vi "TEST_Setup_ExcitsEjects.vi"() -> ()   [LabVIEW 2017]
uses:
  controls/EXCIT_Form_Selector.ctl
  controls/EXCIT_Table.ctl
panel:
  in  "EXCIT Table":T1={"Number of Excits"=0, "Number of Ejects"=0, "Sampling Frequency"=0.0, "Waveforms Table"=[["Excit1", "name", "Swift", "0.5", "1200", "70", "150", "550", "0", "0", "0"]]}
  out "Variant out":variant
  in  "Variant":variant
  out "error out":errorcluster caption="sortie d'erreur"
  in  "error in (no error)":errorcluster
  in  "Excit Form":T2=enum."Swift"
  out "Excitation Signal":T3(graph)
  in  "Fs":dbl=1.0 caption="Sampling Frequency (MHz)" min=1.0 max=100.0
  out "Wfm table":cluster{"Excits Table":string[][]}
  in  "Excit Sandbox":i32(listbox)
  in  "Ejects":u32
  in  "Excits":u32
  in  "Generate":bool
  in  "Update":bool
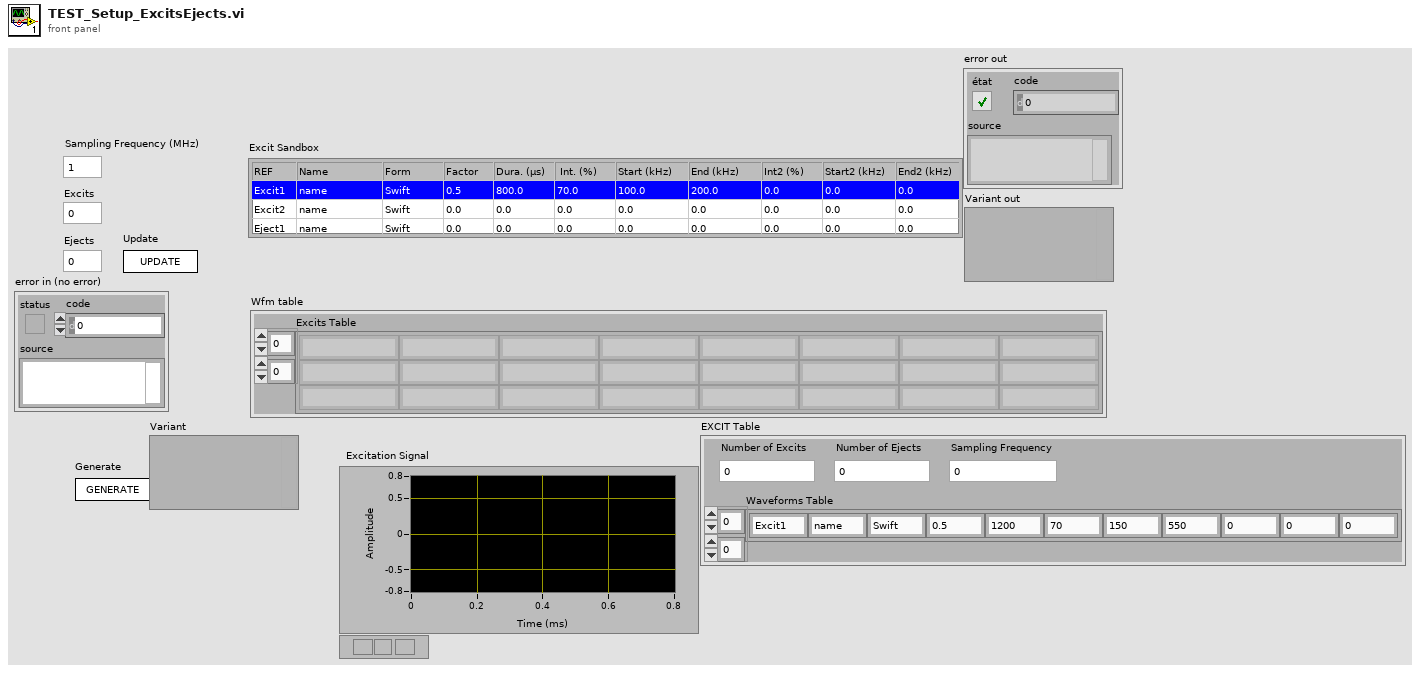
[diagram p1: front panel]
types:
  T1 = typedef "EXCIT_Table.ctl" = cluster{"Number of Excits":u16, "Number of Ejects":u16, "Sampling Frequency":dbl, "Waveforms Table":string[][]}
  T2 = typedef "EXCIT_Form_Selector.ctl" = enum16{"Sinus", "Chirp", "Swift", "TwoSwift", "Ramp"}
  T3 = cluster{"X Time":dbl[], "Signal Excitation":dbl[]}
  T4 = enum16{"Sinus", "Chirp", "Swift", "TwoSwift", "Ramp"}
  T5 = typedef "LVRowAndColumnTypeDef.ctl" = cluster{"Row":i32, "Column":i32}
  T6 = typedef "LVPoint32TypeDef.ctl" = cluster{"Horizontal":i32, "Vertical":i32}
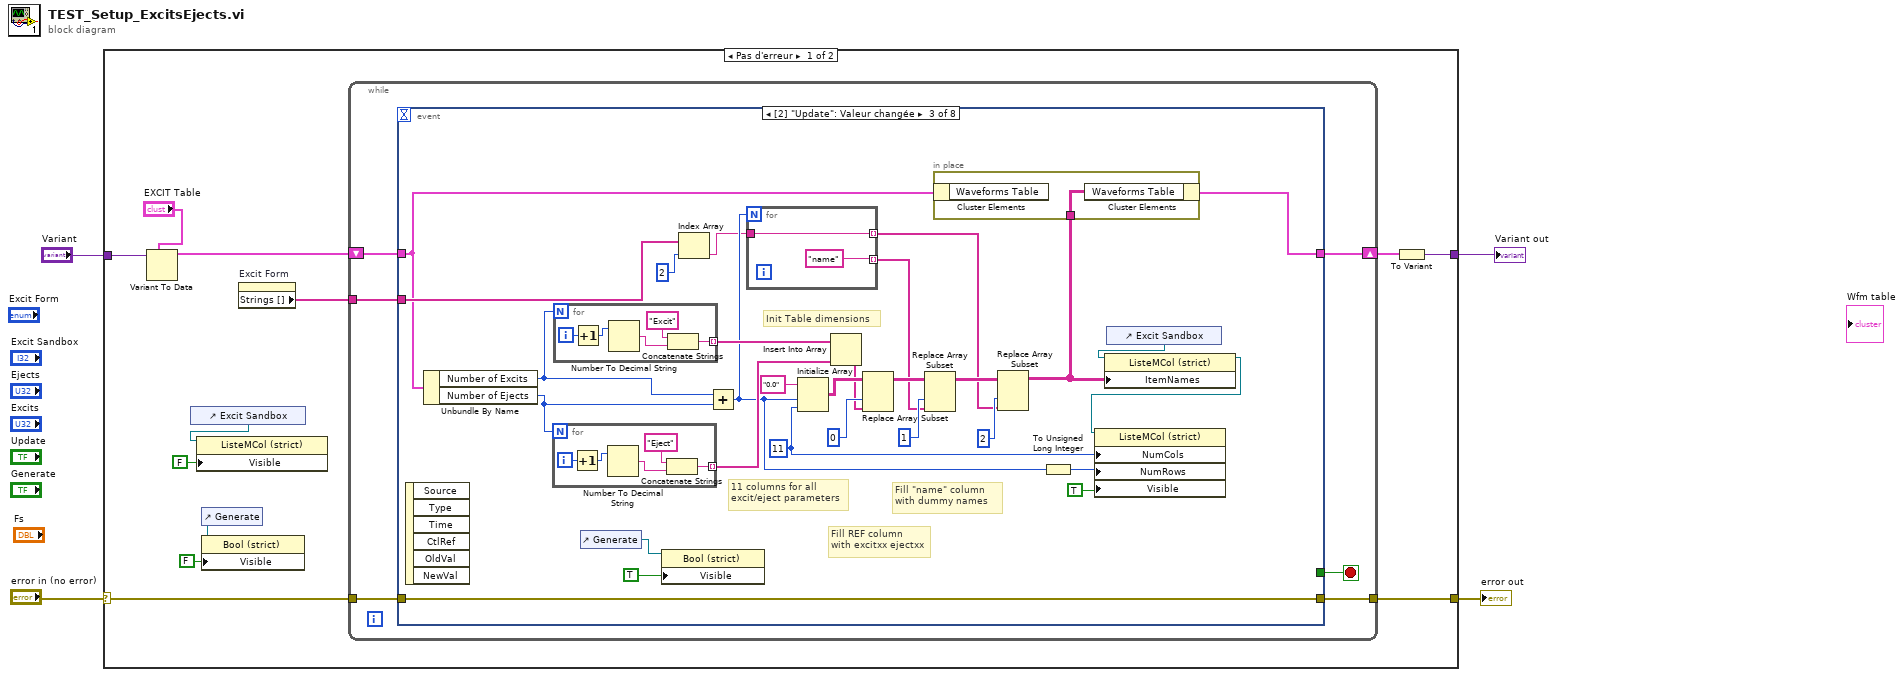
[diagram p0: block diagram]
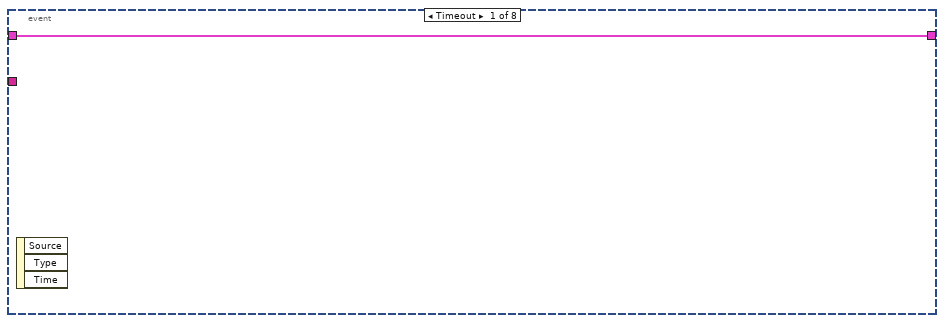
[diagram p2: hidden frame]
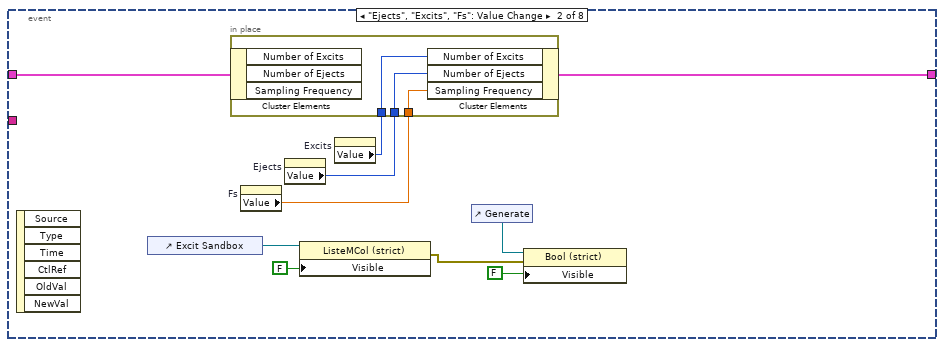
[diagram p3: hidden frame]
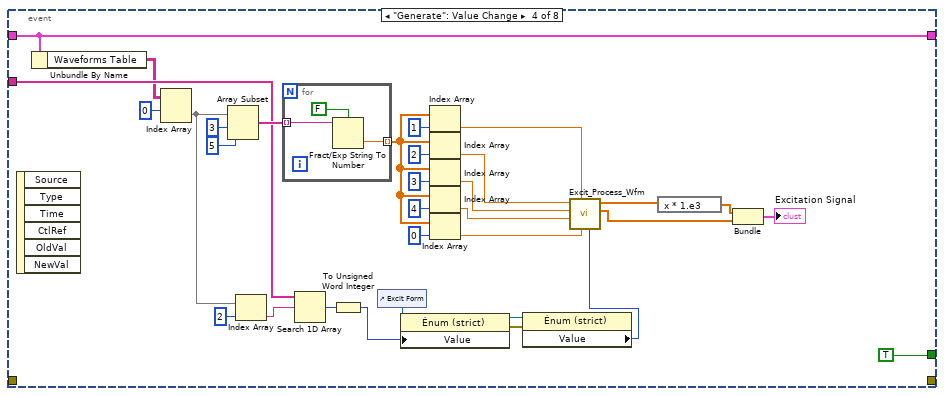
[diagram p4: hidden frame]
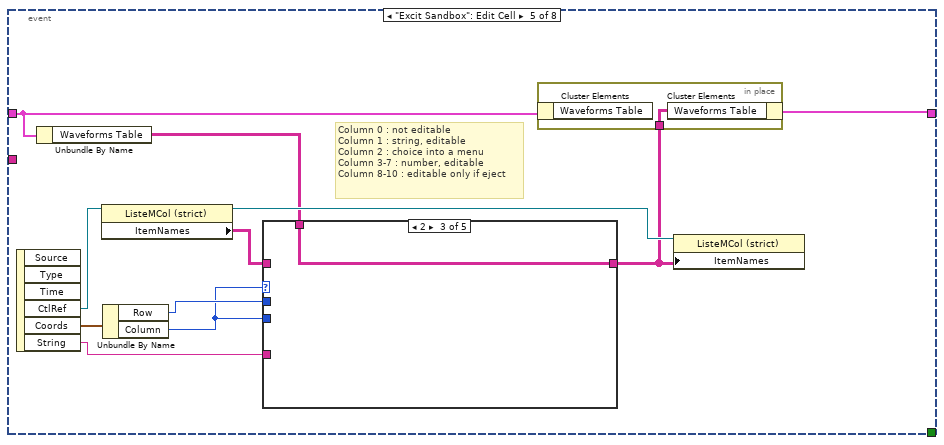
[diagram p5: hidden frame]
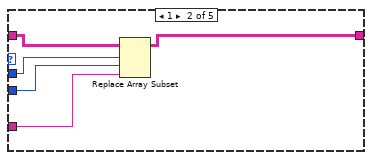
[diagram p7: hidden frame]
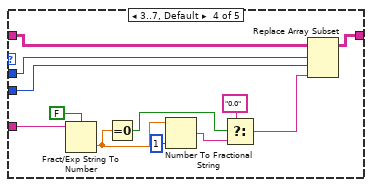
[diagram p8: hidden frame]
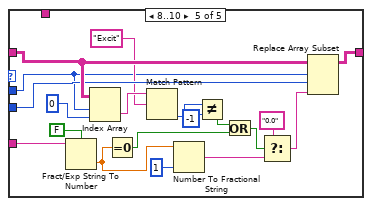
[diagram p9: hidden frame]
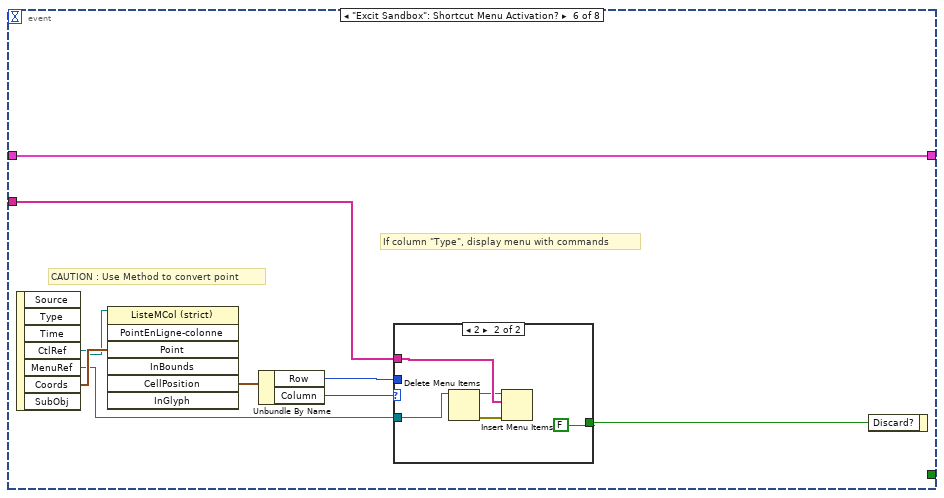
[diagram p10: hidden frame]
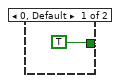
[diagram p11: hidden frame]
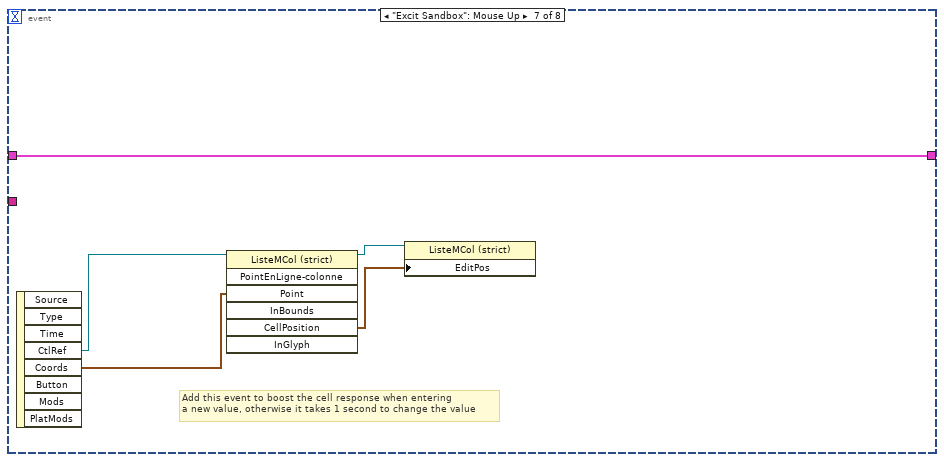
[diagram p12: hidden frame]
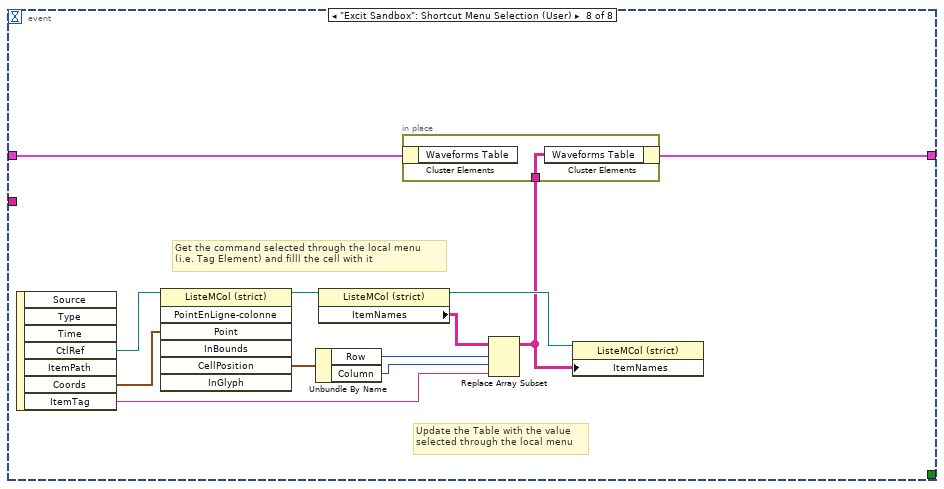
[diagram p13: hidden frame]
diagram:
  n1 = case shown="Pas d'erreur" "error in (no error)" {
    selector: "error in (no error)" -> [w6 _]
    tunnel: "Variant" -> [w11 _]
    tunnel: [w7 _] -> w2
    tunnel: [w5 _] -> w1
    frame No Error {
      n2 = Variant To Data(type="EXCIT Table", Variant=w11) -> (data=w9:T1)  [unwired: 1 in, 1 out]
      n3 = control-ref of="Excit Sandbox"() -> (w14:refnum<vi>)
      n4 = property class="ListeMCol (strict)"(reference=w14, "Visible"=FALSE) -> ()  [unwired: 1 in, 2 out]
      n5 = control-ref of="Generate"() -> (w16:refnum<vi>)
      n6 = property class="Bool (strict)"(reference=w16, "Visible"=FALSE) -> ()  [unwired: 1 in, 2 out]
      n7 = property on="Excit Form" class="Énum (strict)"() -> ("Strings []"=w12:string[])  [unwired: 2 in, 2 out]
      n8 = while {
        tunnel: w12 -> [w21]
        shift-right: [w19] -> w8
        shift-left: w9 -> [w20]
        tunnel: w6 -> [w18]
        tunnel: [w17] -> w5
        stop <- w22 stop-if-true
        n9 = event shown="[2] \"Update\": Valeur changée" {
          selector: _ -> [_ _ _ _ _ _ _ _]
          dyn-events: _ -> [_ _ _ _ _ _ _ _]
          timeout: _ -> [_ _ _ _ _ _ _ _]
          tunnel: [_ _ _ TRUE _ _ _ _] -> w22
          tunnel: w21 -> [_ _ w52 w91 _ w167 _ _]
          tunnel: w20 -> [w23 w28 w40 w79 w116 w164 w179 w186]
          tunnel: [w23 w24 w38 w79 w114 w164 w179 w184] -> w19
          tunnel: w18 -> [_ _ w37 _ _ _ _ _]
          tunnel: [_ _ w37 _ _ _ _ _] -> w17
          event Timeout {
            n10 = event-data() -> ()  [unwired: 1 in, 3 out]
          }
          event "Ejects", "Excits", "Fs": Value Change {
            n11 = event-data() -> ()  [unwired: 1 in, 6 out]
            n12 = control-ref of="Excit Sandbox"() -> (w30:refnum<vi>)
            n13 = property on="Fs" class="NumNb (strict)"() -> ("Value"=w25:dbl)  [unwired: 2 in, 2 out]
            n14 = property on="Ejects" class="NumNb (strict)"() -> ("Value"=w26:u32)  [unwired: 2 in, 2 out]
            n15 = property class="ListeMCol (strict)"(reference=w30, "Visible"=FALSE) -> (error out=w29:errorcluster)  [unwired: 1 in, 1 out]
            n16 = property on="Excits" class="NumNb (strict)"() -> ("Value"=w27:u32)  [unwired: 2 in, 2 out]
            n17 = in-place {
              in-place-border: w27 -> [w36]
              in-place-border: w26 -> [w35]
              in-place-border: w25 -> [w34]
              n18 = in-place-cluster #1(w28) -> ()  [unwired: 3 out]
              n19 = in-place-cluster #1("Number of Excits"=w36, "Number of Ejects"=w35, "Sampling Frequency"=w34) -> (w24:T1)
            }
            n20 = control-ref of="Generate"() -> (w32:refnum<vi>)
            n21 = property class="Bool (strict)"(reference=w32, error in=w29, "Visible"=FALSE) -> ()  [unwired: 2 out]
          }
          event "Update": Value Change {
            w58 = 11 ("taille de la dimension")
            # "11 columns for all\nexcit/eject parameters"
            # "Fill \"name\" column\nwith dummy names"
            # "Fill REF column\nwith excitxx ejectxx"
            # "Init Table dimensions"
            n22 = event-data() -> ()  [unwired: 1 in, 6 out]
            n23 = Unbundle By Name(w40) -> ("Number of Excits"=w42:u16, "Number of Ejects"=w41:u16)
            n24 = for {
              N: w41 -> [_]
              tunnel: [w75] -> w48 mode=indexing
              i -> [w78]
              n25 = Increment(x=w78) -> (x+1=w74:i32)
              n26 = Number To Decimal String(number=w74) -> (decimal integer string=w77:string)  [unwired: 1 in]
              n27 = Concatenate Strings("Eject" ("chaîne"), w77) -> (w75:string)
            }
            n28 = for {
              N: w42 -> [_]
              tunnel: [w70] -> w49 mode=indexing
              i -> [w73]
              n29 = Increment(x=w73) -> (x+1=w69:i32)
              n30 = Number To Decimal String(number=w69) -> (decimal integer string=w72:string)  [unwired: 1 in]
              n31 = Concatenate Strings("Excit" ("chaîne"), w72) -> (w70:string)
            }
            n32 = control-ref of="Generate"() -> (w64:refnum<vi>)
            n33 = property class="Bool (strict)"(reference=w64, "Visible"=TRUE) -> ()  [unwired: 1 in, 2 out]
            n34 = Index Array(array=w52, index=2 ("indice")) -> (element=w45:string)
            n35 = Add(x=w42, y=w41) -> (x+y=w46:u16)
            n36 = for {
              N: w46 -> [_]
              tunnel: ["name" ("chaîne")] -> w44 mode=indexing
              tunnel: w45 -> [w67]
              tunnel: [w67] -> w43 mode=indexing
            }
            n37 = Initialize Array("0.0" ("élément"), w46, w58) -> (w57:string[][])
            n38 = Insert Into Array(array=w49, new element=w48) -> (w47:string[])  [unwired: 1 in]
            n39 = Replace Array Subset(array=w57, new element=w47, index (col)=0 ("indice désactivé (col)")) -> (w55:string[][])  [unwired: 1 in]
            n40 = Replace Array Subset(array=w55, new element=w44, index (col)=1 ("indice désactivé (col)")) -> (w53:string[][])  [unwired: 1 in]
            n41 = Replace Array Subset(array=w53, new element=w43, index (col)=2 ("indice désactivé (col)")) -> (w39:string[][])  [unwired: 1 in]
            n42 = in-place {
              in-place-border: w39 -> [w66]
              n43 = in-place-cluster #2(w40) -> ()  [unwired: 1 out]
              n44 = in-place-cluster #2("Waveforms Table"=w66) -> (w38:T1)
            }
            n45 = To Unsigned Long Integer(number=w46) -> (unsigned 32bit integer=w63:u32)
            n46 = control-ref of="Excit Sandbox"() -> (w60:refnum<vi>)
            n47 = property class="ListeMCol (strict)"(reference=w60, "ItemNames"=w39) -> (reference out=w61:refnum<vi>)  [unwired: 1 in, 1 out]
            n48 = property class="ListeMCol (strict)"(reference=w61, "NumCols"=w58, "NumRows"=w63, "Visible"=TRUE) -> ()  [unwired: 1 in, 2 out]
          }
          event "Generate": Value Change {
            n49 = event-data() -> ()  [unwired: 1 in, 6 out]
            n50 = Unbundle By Name(w79) -> ("Waveforms Table"=w80:string[][])
            n51 = Index Array(array=w80, index (row)=0 ("indice (ligne)")) -> (element=w94:string[])  [unwired: 1 in]
            n52 = Array Subset(array=w94, index=3 ("indice"), length=5 ("longueur")) -> (w106:string[])
            n53 = Index Array(array=w94, index=2 ("indice")) -> (element=w92:string)
            n54 = for {
              tunnel: w106 -> [w113] mode=indexing
              tunnel: [w111] -> w105 mode=indexing
              n55 = Fract/Exp String To Number(use system decimal point (T)=FALSE ("utiliser le séparateur décimal du système (V)"), string=w113) -> (number=w111:dbl)  [unwired: 2 in, 1 out]
            }
            n56 = Search 1D Array(1D array=w91, element=w92) -> (index of element=w84:i32)  [unwired: 1 in]
            n57 = To Unsigned Word Integer(number=w84) -> (unsigned 16bit integer=w83:u16)
            n58 = control-ref of="Excit Form"() -> (w81:refnum<vi>)
            n59 = property class="Énum (strict)"(reference=w81, "Value"=w83) -> (reference out=w86:refnum<vi>, error out=w85:errorcluster)  [unwired: 1 in]
            n60 = Index Array(array=w105, index=1 ("indice")) -> (element=w95:dbl)
            n61 = Index Array(array=w105, index=2 ("indice")) -> (element=w97:dbl)
            n62 = Index Array(array=w105, index=3 ("indice")) -> (element=w99:dbl)
            n63 = Index Array(array=w105, index=4 ("indice")) -> (element=w101:dbl)
            n64 = Index Array(array=w105, index=0 ("indice")) -> (element=w103:dbl)
            n65 = property class="Énum (strict)"(reference=w86, error in=w85) -> ("Value"=w82:T4)  [unwired: 2 out]
            n66 = call "Excit_Process_Wfm.vi"("Excit Form"=w82, "Factor"=w103, "Duration (µs)"=w95, "End Frequency (kHz)"=w101, "Start Frequency (kHz)"=w99, "Amplitude (%)"=w97) -> ("Signal Excitation"=w88:dbl[], "X Time"=w89:dbl[])  [unwired: 1 in, 2 out]
            n67 = expression code="x * 1.e3"(w89) -> (w90:dbl[])
            n68 = Bundle("X Time"=w90, "Signal Excitation"=w88) -> (→"Excitation Signal":T3)  [unwired: 1 in]
          }
          event "Excit Sandbox": Edit Cell {
            # "Column 0 : not editable\nColumn 1 : string, editable\nColumn 2 : choice into a menu\nColumn 3-7 : number, editable\nColumn 8-10 : editable only if eject"
            n69 = event-data() -> ("CtlRef"=w124:refnum<vi>, "Coords"=w120:T5, "String"=w123:string)  [unwired: 1 in, 3 out]
            n70 = Unbundle By Name(w116) -> ("Waveforms Table"=w117:string[][])
            n71 = property class="ListeMCol (strict)"(reference=w124) -> (reference out=w118:refnum<vi>, "ItemNames"=w122:string[][])  [unwired: 1 in, 1 out]
            n72 = Unbundle By Name(w120) -> ("Row"=w121:i32, "Column"=w119:i32)
            n73 = case shown="2" w119 {
              tunnel: w123 -> [_ w131 _ w144 w163]
              tunnel: w122 -> [_ w128 _ w134 w155]
              tunnel: w121 -> [_ w127 _ w133 w145]
              tunnel: w119 -> [_ w130 _ w143 w154]
              tunnel: [w126 w129 w132 w142 w162] -> w115
              tunnel: w117 -> [w126 _ w132 _ _]
              frame 0 {
              }
              frame 1 {
                n74 = Replace Array Subset(array=w128, new element=w131, index (row)=w127, index (col)=w130) -> (w129:string[][])
              }
              frame 2 {
              }
              frame 3..7, Default {
                n75 = Fract/Exp String To Number(use system decimal point (T)=FALSE ("utiliser le séparateur décimal du système (V)"), string=w144) -> (number=w138:dbl)  [unwired: 2 in, 1 out]
                n76 = Equal To 0?(x=w138) -> (x = 0?=w135:bool)
                n77 = Number To Fractional String(number=w138, precision (6)=i16 1 ("précision (6)")) -> (F-format string=w136:string)  [unwired: 2 in]
                n78 = Select(t="0.0", s=w135, f=w136) -> (s? t:f=w140:string)
                n79 = Replace Array Subset(array=w134, new element=w140, index (row)=w133, index (col)=w143) -> (w142:string[][])
              }
              frame 8..10 {
                n80 = Fract/Exp String To Number(use system decimal point (T)=FALSE ("utiliser le séparateur décimal du système (V)"), string=w163) -> (number=w158:dbl)  [unwired: 2 in, 1 out]
                n81 = Index Array(array=w155, index (row)=w145, index (col)=0 ("indice désactivé (col)")) -> (element=w152:string)
                n82 = Equal To 0?(x=w158) -> (x = 0?=w149:bool)
                n83 = Match Pattern(string=w152, regular expression="Excit" ("expression régulière")) -> (offset past match=w148:i32)  [unwired: 1 in, 3 out]
                n84 = Number To Fractional String(number=w158, precision (6)=i16 1 ("précision (6)")) -> (F-format string=w156:string)  [unwired: 2 in]
                n85 = Not Equal?(x=w148, y=-1) -> (x != y?=w146:bool)
                n86 = Or(x=w146, y=w149) -> (x .or. y?=w150:bool)
                n87 = Select(t="0.0", s=w150, f=w156) -> (s? t:f=w160:string)
                n88 = Replace Array Subset(array=w155, new element=w160, index (row)=w145, index (col)=w154) -> (w162:string[][])
              }
            }
            n89 = in-place {
              in-place-border: w115 -> [w125]
              n90 = in-place-cluster #3(w116) -> ()  [unwired: 1 out]
              n91 = in-place-cluster #3("Waveforms Table"=w125) -> (w114:T1)
            }
            n92 = property class="ListeMCol (strict)"(reference=w118, "ItemNames"=w115) -> ()  [unwired: 1 in, 2 out]
          }
          event "Excit Sandbox": Shortcut Menu Activation? {
            # "If column \"Type\", display menu with commands"
            # "CAUTION : Use Method to convert point"
            n93 = event-data() -> ("CtlRef"=w165:refnum<vi>, "MenuRef"=w168:refnum<k9>, "Coords"=w169:T6)  [unwired: 1 in, 4 out]
            n94 = invoke class="ListeMCol (strict)" method="PointEnLigne-colonne"(reference=w165, "Point"=w169) -> ("CellPosition"=w172:T5)  [unwired: 5 in, 6 out]
            n95 = Unbundle By Name(w172) -> ("Row"=w170:i32, "Column"=w171:i32)
            n96 = case shown="2" w171 {
              tunnel: [TRUE FALSE] -> w166
              tunnel: w168 -> [_ w178]
              tunnel: w170 -> [_ _]
              tunnel: w167 -> [_ w176]
              frame 0, Default {
              }
              frame 2 {
                n97 = Delete Menu Items(9:w178) -> (0:w175:errorcluster, 3:w174:refnum<k9>)  [unwired: 3 in]
                n98 = Insert Menu Items(6:w175, 8:w176, 9:w174) -> ()  [unwired: 3 in, 3 out]
              }
            }
            n99 = event-data("Discard?"=w166) -> ()  [unwired: 1 in, 1 out]
          }
          event "Excit Sandbox": Mouse Up {
            # "Add this event to boost the cell response when entering\na new value, otherwise it takes 1 second to change the value"
            n100 = event-data() -> ("CtlRef"=w180:refnum<vi>, "Coords"=w181:T6)  [unwired: 1 in, 6 out]
            n101 = invoke class="ListeMCol (strict)" method="PointEnLigne-colonne"(reference=w180, "Point"=w181) -> (reference out=w183:refnum<vi>, "CellPosition"=w182:T5)  [unwired: 5 in, 5 out]
            n102 = property class="ListeMCol (strict)"(reference=w183, "EditPos"=w182) -> ()  [unwired: 1 in, 2 out]
          }
          event "Excit Sandbox": Shortcut Menu Selection (User) {
            # "Update the Table with the value\nselected through the local menu"
            # "Get the command selected through the local menu\n(i.e. Tag Element) and filll the cell with it"
            n103 = event-data() -> ("CtlRef"=w190:refnum<vi>, "Coords"=w191:T6, "ItemTag"=w188:string)  [unwired: 1 in, 4 out]
            n104 = invoke class="ListeMCol (strict)" method="PointEnLigne-colonne"(reference=w190, "Point"=w191) -> (reference out=w194:refnum<vi>, "CellPosition"=w195:T5)  [unwired: 5 in, 5 out]
            n105 = Unbundle By Name(w195) -> ("Row"=w192:i32, "Column"=w189:i32)
            n106 = property class="ListeMCol (strict)"(reference=w194) -> (reference out=w193:refnum<vi>, "ItemNames"=w187:string[][])  [unwired: 1 in, 1 out]
            n107 = Replace Array Subset(array=w187, new element=w188, index (row)=w192, index (col)=w189) -> (w185:string[][])
            n108 = in-place {
              in-place-border: w185 -> [w196]
              n109 = in-place-cluster #4(w186) -> ()  [unwired: 1 out]
              n110 = in-place-cluster #4("Waveforms Table"=w196) -> (w184:T1)
            }
            n111 = property class="ListeMCol (strict)"(reference=w193, "ItemNames"=w185) -> ()  [unwired: 1 in, 2 out]
          }
        }
      }
      n112 = To Variant(anything=w8) -> (Variant=w7:variant)
    }
    frame Error {
    }
  }
  "error out" <- w1
  "Variant out" <- w2
